vi "Send CamTestGetEvntsResponse.vi"(7 "Message Priority (Normal)":T8=enum."Normal", 8 "error in (no error)":errorcluster, 10 "CameraTestingEvnt":T1, 11 "Message Enqueuer":refnum<class "Message Enqueuer.lvclass">) -> (0 "error out":errorcluster, 3 "Message Enqueuer out":refnum<class "Message Enqueuer.lvclass">)   [LabVIEW 2020, in "ICameraTestingUI.lvlib" / "CamTestGetEvntsResponse Msg.lvclass"]
doc: "This VI sends the message to an actor."
uses:
  CamTestGetEvntsResponse Msg.lvclass
  <vilib>/ActorFramework/Message Enqueuer/Message Enqueuer.lvclass
  <vilib>/ActorFramework/Message Enqueuer/Message Priority.ctl
  ICameraTesting/TypeDef/Events.ctl
  Camera/ICamera/TypeDef/SnapInfo.ctl
  ICameraTesting/TypeDef/FrameRateValReceived.ctl
  ICameraTesting/TypeDef/ImgTypeValReceived.ctl
  ICameraTesting/TypeDef/ResolutionValReceived.ctl
  ICameraTesting/TypeDef/VideoOptCodesUpdated.ctl
  ICameraTesting/TypeDef/VideoOptionsInfo.ctl
  ICameraTesting/TypeDef/StatusUpdated.ctl
  ICameraTesting/TypeDef/StatusRecord.ctl
  ICameraTesting/TypeDef/VideoBufferUpdate.ctl
  C:/Program Files (x86)/National Instruments/LabVIEW 2020/vi.lib/ActorFramework/Message/Message.lvclass
  CamTestGetEvntsResponse Msg.lvclass/CamTestGetEvntsResponse Msg.ctl
  <vilib>/ActorFramework/Message Enqueuer/Message Enqueuer.lvclass/Message Enqueuer.ctl
  <vilib>/ActorFramework/Message Priority Queue/Priority Enqueue.vi
  Camera/ICamera/TypeDef/ICamera_typedef.lvlib
  ICameraTesting/TypeDef/ICameraTesting_typedef.lvlib
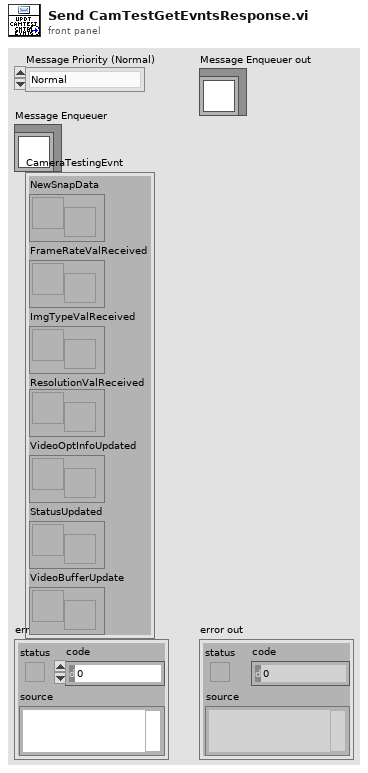
[diagram p1: front panel]
types:
  T1 = typedef "ICameraTesting_typedef.lvlib/Events.ctl" = cluster{"NewSnapData":refnum<user-event>, "FrameRateValReceived":T2, "ImgTypeValReceived":T3, "ResolutionValReceived":T4, "VideoOptInfoUpdated":T5, "StatusUpdated":T6, "VideoBufferUpdate":T7}
  T2 = typedef "ICameraTesting_typedef.lvlib/FrameRateValReceived.ctl" = refnum<user-event>
  T3 = typedef "ICameraTesting_typedef.lvlib/ImgTypeValReceived.ctl" = refnum<user-event>
  T4 = typedef "ICameraTesting_typedef.lvlib/ResolutionValReceived.ctl" = refnum<user-event>
  T5 = typedef "ICameraTesting_typedef.lvlib/VideoOptCodesUpdated.ctl" = refnum<user-event>
  T6 = typedef "ICameraTesting_typedef.lvlib/StatusUpdated.ctl" = refnum<user-event>
  T7 = typedef "ICameraTesting_typedef.lvlib/VideoBufferUpdate.ctl" = refnum<user-event>
  T8 = typedef "Actor Framework.lvlib/Message Enqueuer.lvclass/Message Priority.ctl" = enum16{"Low", "Normal", "High"}
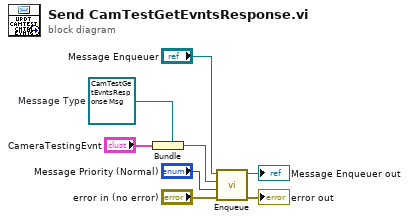
[diagram p0: block diagram]
diagram:
  w5 = refnum<class "CamTestGetEvntsResponse Msg.lvclass"> refnum  # Message Type
  n1 = Bundle(cluster=w5, "CameraTestingEvnt") -> (w4:refnum<class "CamTestGetEvntsResponse Msg.lvclass">)
  n2 = call <vilib>:"Enqueue.vi"("error in (no error)"="error in (no error)", "Message Priority (Normal)"="Message Priority (Normal)", "Message"=w4, "Message Enqueuer in"="Message Enqueuer") -> ("error out"=→"error out":errorcluster, "Message Enqueuer out"=→"Message Enqueuer out":refnum<class "Message Enqueuer.lvclass">)  [unwired: 6 in]
